vi "Open DSF Configuration Data.vi"(8 "error in (no error)":errorcluster, 10 "create file if necessary (T)":bool=TRUE, 11 "dsf configuration file path":path) -> (0 "error out":errorcluster, 2 "file created?":bool, 3 "dsf refnum":T2, 4 "version":T1)   [LabVIEW 2017, in "DSF Configuration API.lvlib"]
doc: "Opens a reference to the configuration data found in a platform-independent configuration file."
uses:
  DSF Configuration API.lvlib
  Controls/DSF Config Data RefNum.ctl
  Controls/DSF Version Info.ctl
  Private/Controls/Session/DSF Config Data.ctl
  Private/Controls/DSF File Format/Internal.DSF Configuration.ctl
  Private/Controls/DSF File Format/Internal.DSF Plugin with ID.ctl
  Private/Controls/DSF File Format/Internal.DSF Plugin Info.ctl
  Controls/DSF Timing Info.ctl
  Private/Controls/DSF File Format/Internal.DSF Group with ID.ctl
  Private/Controls/DSF File Format/Internal.DSF Group Info.ctl
  Private/Controls/DSF File Format/Internal.DSF Transfer with ID.ctl
  Private/Controls/DSF File Format/Internal.DSF Transfer Info.ctl
  Private/Controls/DSF File Format/Internal.DSF Channel with ID.ctl
  Private/Controls/DSF File Format/Internal.DSF Channel Info.ctl
  Private/Controls/DSF File Format/Internal.DSF Settings with ID.ctl
  Private/Controls/DSF File Format/Internal.DSF Settings Info.ctl
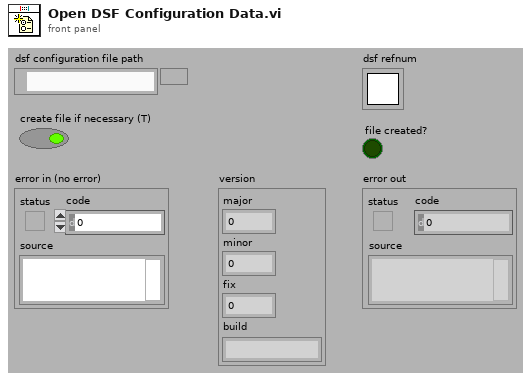
[diagram p1: front panel]
types:
  T1 = typedef "DSF Configuration API.lvlib/DSF Version Info.ctl" = cluster{"major":u32, "minor":u32, "fix":u32, "build":string}
  T2 = typedef "DSF Configuration API.lvlib/DSF Config Data RefNum.ctl" = refnum<k1>
  T3 = typedef "DSF Configuration API.lvlib/DSF Config Data.ctl" = cluster{"dsf configuration":T4, "path":path, "dirty":bool}
  T4 = typedef "DSF Configuration API.lvlib/Internal.DSF Configuration.ctl" = cluster{"dsfversion":T1, "version":T1, "plugins":T5[], "groups":T8[], "transfers":T10[], "channels":T12[], "settings":T14[]}
  T5 = typedef "DSF Configuration API.lvlib/Internal.DSF Plugin with ID.ctl" = cluster{"id":string, "values":T6}
  T6 = typedef "DSF Configuration API.lvlib/Internal.DSF Plugin Info.ctl" = cluster{"type":string, "timing":T7, "group ids":string[], "settings id":string}
  T7 = typedef "DSF Configuration API.lvlib/DSF Timing Info.ctl" = cluster{"priority":i32, "decimation":i32, "offset":i32}
  T8 = typedef "DSF Configuration API.lvlib/Internal.DSF Group with ID.ctl" = cluster{"id":string, "values":T9}
  T9 = typedef "DSF Configuration API.lvlib/Internal.DSF Group Info.ctl" = cluster{"direction":i32, "timing":T7, "transfer ids":string[], "settings id":string}
  T10 = typedef "DSF Configuration API.lvlib/Internal.DSF Transfer with ID.ctl" = cluster{"id":string, "values":T11}
  T11 = typedef "DSF Configuration API.lvlib/Internal.DSF Transfer Info.ctl" = cluster{"byte order":i32, "channel ids":string[], "settings id":string}
  T12 = typedef "DSF Configuration API.lvlib/Internal.DSF Channel with ID.ctl" = cluster{"id":string, "values":T13}
  T13 = typedef "DSF Configuration API.lvlib/Internal.DSF Channel Info.ctl" = cluster{"count":i32, "offset":i32, "data type":i32, "resource path":string, "settings id":string}
  T14 = typedef "DSF Configuration API.lvlib/Internal.DSF Settings with ID.ctl" = cluster{"id":string, "values":T15}
  T15 = typedef "DSF Configuration API.lvlib/Internal.DSF Settings Info.ctl" = cluster{"key":string, "value":string}[]
  T16 = typedef "DSF Configuration API.lvlib/DSF Configuration Reference.ctl" = refnum<data-value>
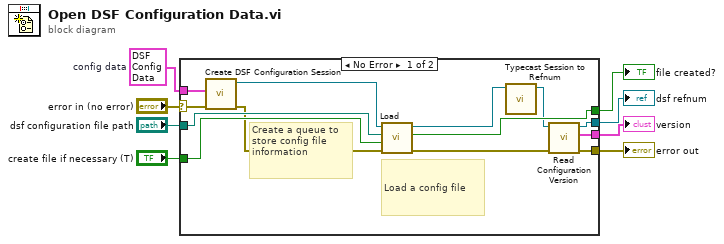
[diagram p0: block diagram]
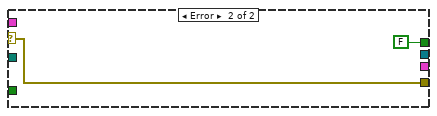
[diagram p2: hidden frame]
diagram:
  w2 = T3 {"dsf configuration"={"dsfversion"={"major"=0, "minor"=0, "fix"=0, "build"=""}, "version"={"major"=0, "minor"=0, "fix"=0, "build"=""}, "plugins"=[], "groups"=[], "transfers"=[], "channels"=[], "settings"=[]}, "path"=path "", "dirty"=FALSE}  # config data
  n1 = case shown="No Error" "error in (no error)" {
    selector: "error in (no error)" -> [w17 w23]
    tunnel: "dsf configuration file path" -> [w21 _]
    tunnel: "create file if necessary (T)" -> [w20 _]
    tunnel: [w18 FALSE ("file created?")] -> w4
    tunnel: [w13 w23] -> w5
    tunnel: w2 -> [w9 _]
    tunnel: [w11 _] -> w3
    tunnel: [w10 _] -> w1
    frame No Error {
      # "Load a config file"
      # "Create a queue to store config file information"
      n2 = call "Create DSF Configuration Session.vi"("error in (no error)"=w17, "config data"=w9) -> ("error out"=w16:errorcluster, "DSF Configuration Session out"=w14:T16)  [unwired: 8 in]
      n3 = call "Load.vi"("error in (no error)"=w16, "create file if necessary? (T)"=w20, "configuration file path"=w21, "DSF Configuration Reference in"=w14) -> ("error out"=w19:errorcluster, "file created?"=w18:bool, "DSF Configuration Reference out"=w15:T16)  [unwired: 5 out]
      n4 = call "Typecast Session to Refnum.vi"("DSF Configuration Reference in"=w15) -> ("dsf refnum out"=w12:T2)  [unwired: 10 in]
      n5 = call "Read Configuration Version.vi"("error in (no error)"=w19, "dsf refnum"=w12) -> ("error out"=w13:errorcluster, "version"=w10:T1, "dsf refnum out"=w11:T2)  [unwired: 7 in]
    }
    frame Error {
    }
  }
  "error out" <- w5
  "file created?" <- w4
  "dsf refnum" <- w3
  "version" <- w1
